vi "conversion_rad_to_deg.vi"(1 "Angle (rad)":dbl) -> (0 "Angle (deg)":dbl)   [LabVIEW 2021]
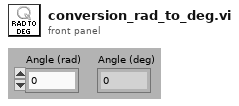
[diagram p1: front panel]
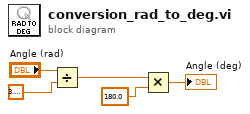
[diagram p0: block diagram]
diagram:
  n1 = Divide(x="Angle (rad)", y=3.141592653589793) -> (x/y=w5:dbl)
  n2 = Multiply(x=w5, y=180.0) -> (x*y=→"Angle (deg)":dbl)
